vi "Wyznaczanie prędkości kół i odległości do punktu docelowego.vi"(7 "Odl. pkt. docelowego od startu[m]":cluster{"X/E [m]":dbl, "Y/N [m]":dbl} caption="Odległość punktu docelowego od startu [m]", 8 "Azymut robota [stopnie]":dbl, 9 "Odległość robota od startu":cluster{"X[m]":dbl, "Y[m]":dbl}, 11 "fuzzy system in":T1 {"user MF interpolating polynomials"."coa_x(y) coeff" format="%.4g"; "user MF interpolating polynomials"."Area(y) coeff" format="%.4g"; "user MF interpolating polynomials"."X(y) coeff" format="%.4g"; "user MF interpolating polynomials"."Y(x) coeff" format="%.4g"; "user MF interpolating polynomials"."Y" format="%.4g"; "user MF interpolating polynomials"."X" format="%.4g"; "defuzzification method" items=["Center of Area", "Modified Center of Area", "Center of Sums", "Center of Maximum", "Mean of Maximum"]; "rules"."consequents"."Var Index" min=0; "rules"."consequents"."Cond" items=["=", "!="]; "rules"."consequents"."MF Index" min=0; "rules"."antecedents"."Var Index" min=0; "rules"."antecedents"."Cond" items=["=", "!="]; "rules"."antecedents"."MF Index" min=0; "rules"."consequent implication" items=["Minimum", "Product"]; "rules"."antecedent connective" items=["AND (Minimum)", "AND (Product)", "OR (Maximum)", "OR (Probabilistic)"]; "output variables"."MFs"."shape" items=["Triangle", "Trapezoid", "Singleton", "Sigmoid", "Gaussian", "User-Defined"]; "input variables"."MFs"."shape" items=["Triangle", "Trapezoid", "Singleton", "Sigmoid", "Gaussian", "User-Defined"]}) -> (1 "Prędkości kół":cluster{"prawe [rad/s]":dbl, "lewe [rad/s]":dbl}, 3 "Odległość do punktu zadanego [m]":dbl)   [LabVIEW 2012, in "Biblioteka moduł map v3.lvlib" / "Pomocnicze.lvlib"]
doc: "Wyznacza na podstawie odległości i odchylenia kątowego robota od kierunku docelowego wartości sterujących prędkościami kół."
uses:
  Pomocnicze.lvlib
  <vilib>/addons/Fuzzy Logic/TypeDefs/FL System.ctl
  <vilib>/addons/Fuzzy Logic/TypeDefs/FL Variable.ctl
  <vilib>/addons/Fuzzy Logic/TypeDefs/FL Membership Function.ctl
  <vilib>/addons/Fuzzy Logic/TypeDefs/FL Membership Function Shape.ctl
  <vilib>/addons/Fuzzy Logic/TypeDefs/FL Rule.ctl
  <vilib>/addons/Fuzzy Logic/TypeDefs/FL Antecedent.ctl
  <vilib>/addons/Fuzzy Logic/TypeDefs/FL Modifier.ctl
  <vilib>/addons/Fuzzy Logic/TypeDefs/FL Antecedent Connective.ctl
  <vilib>/addons/Fuzzy Logic/TypeDefs/FL Consequent.ctl
  <vilib>/addons/Fuzzy Logic/TypeDefs/FL Consequent Implication.ctl
  <vilib>/addons/Fuzzy Logic/TypeDefs/FL Defuzzification.ctl
  <vilib>/addons/Fuzzy Logic/TypeDefs/FL Interpolating polynomials.ctl
  <vilib>/addons/Fuzzy Logic/FL Fuzzy Controller (MIMO).vi
  <vilib>/addons/Fuzzy Logic/NI_Fuzzy_Logic_API.lvlib
  Matematyczne/Matematyczne.lvlib
panel:
  # "IF"
  # "THEN"
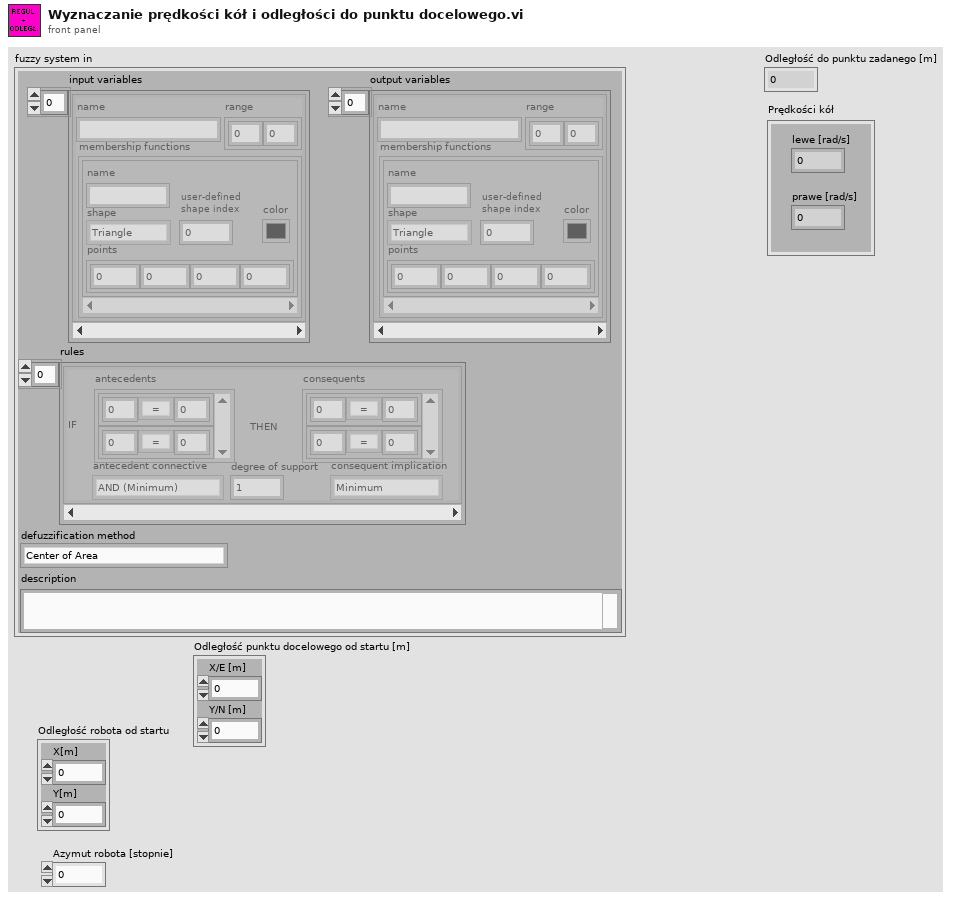
[diagram p1: front panel]
types:
  T1 = typedef "NI_Fuzzy_Logic_API.lvlib/FL System.ctl" = cluster{"input variables":T2[], "output variables":T2[], "rules":T5[], "defuzzification method":T11, "description":string, "user MF interpolating polynomials":T12[]}
  T2 = typedef "NI_Fuzzy_Logic_API.lvlib/FL Variable.ctl" = cluster{"name":string, "range":dbl[], "MFs":T3[]}
  T3 = typedef "NI_Fuzzy_Logic_API.lvlib/FL Membership Function.ctl" = cluster{"name":string, "shape":T4, "points":dbl[], "color":u32, "user-defined shape index":i32}
  T4 = typedef "NI_Fuzzy_Logic_API.lvlib/FL Membership Function Shape.ctl" = u16
  T5 = typedef "NI_Fuzzy_Logic_API.lvlib/FL Rule.ctl" = cluster{"antecedents":T6[], "antecedent connective":T8, "consequents":T9[], "consequent implication":T10, "degree of support":dbl}
  T6 = typedef "NI_Fuzzy_Logic_API.lvlib/FL Antecedent.ctl" = cluster{"Var Index":i32, "MF Index":i32, "Cond":T7}
  T7 = typedef "NI_Fuzzy_Logic_API.lvlib/FL Modifier.ctl" = u16
  T8 = typedef "NI_Fuzzy_Logic_API.lvlib/FL Antecedent Connective.ctl" = u16
  T9 = typedef "NI_Fuzzy_Logic_API.lvlib/FL Consequent.ctl" = cluster{"Var Index":i32, "MF Index":i32, "Cond":T7}
  T10 = typedef "NI_Fuzzy_Logic_API.lvlib/FL Consequent Implication.ctl" = u16
  T11 = typedef "NI_Fuzzy_Logic_API.lvlib/FL Defuzzification.ctl" = u16
  T12 = typedef "NI_Fuzzy_Logic_API.lvlib/FL Interpolating polynomials.ctl" = cluster{"X":dbl[], "Y":dbl[], "Y(x) coeff":dbl[][], "X(y) coeff":dbl[][], "Area(y) coeff":dbl[][], "coa_x(y) coeff":dbl[][]}
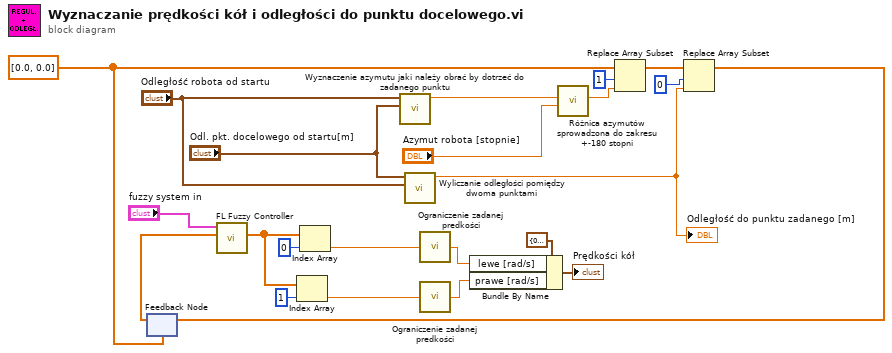
[diagram p0: block diagram]
diagram:
  w1 = dbl[] [0.0, 0.0] ("Odległość i odchylenie kątowe")
  n1 = feedback #1(w1) -> (w2:dbl[])
  n2 = call-poly <vilib>:"FL Fuzzy Controller.vi"("input values"=w2, "fuzzy system in"="fuzzy system in") -> ("output values"=w13:dbl[])  [unwired: 5 in, 4 out]
  n3 = Index Array(array=w13, index=1) -> (element=w5:dbl)
  n4 = Index Array(array=w13, index=0) -> (element=w7:dbl)
  n5 = call "Wyznaczenie azymutu jaki należy obrać by dotrzeć do zadanego punktu.vi"("Położenie końcowe"="Odl. pkt. docelowego od startu[m]", "Położenie aktualne"="Odległość robota od startu") -> ("Azymut"=w21:dbl)  [unwired: 9 in]
  n6 = call "Wyliczanie odległości pomiędzy dwoma punktami.vi"("Polozenie 1"="Odległość robota od startu", "Polozenie in"="Odl. pkt. docelowego od startu[m]") -> ("Numeric"=w17:dbl)  [unwired: 9 in]
  "Odległość do punktu zadanego [m]" <- w17
  n7 = call "Ograniczenie zadanej predkości.vi"("omega [rad/s]"=w7) -> ("Wart. ogr."=w6:dbl)  [unwired: 4 in]
  n8 = call "Ograniczenie zadanej predkości.vi"("omega [rad/s]"=w5) -> ("Wart. ogr."=w4:dbl)  [unwired: 4 in]
  n9 = Bundle By Name(cluster=cluster{"prawe [rad/s]":dbl, "lewe [rad/s]":dbl} {"prawe [rad/s]"=0.0, "lewe [rad/s]"=0.0} ("Prędkości kół"), "lewe [rad/s]"=w6, "prawe [rad/s]"=w4) -> (→"Prędkości kół":cluster{"prawe [rad/s]":dbl, "lewe [rad/s]":dbl})
  n10 = call "Różnica azymutów sprowadzona do zakresu +-180 stopni.vi"("Azymut robota"="Azymut robota [stopnie]", "Azymut - zadany"=w21) -> ("az_z - az_r"=w20:dbl)  [unwired: 9 in]
  n11 = Replace Array Subset(array=w1, new element=w20, index=1) -> (w15:dbl[])
  n12 = Replace Array Subset(array=w15, new element=w17, index=0) -> (w3:dbl[])
  n13 = feedback-in #1(w3) -> ()
